vi "Read UUID.vi"(11 "UniqueName in":refnum<class "UniqueName.lvclass">) -> (2 "UUID":string, 3 "UniqueName out":refnum<class "UniqueName.lvclass">)   [LabVIEW 2014, in "UniqueName.lvlib" / "UniqueName.lvclass"]
uses:
  UniqueName.lvclass
  UniqueName.lvclass/UniqueName.ctl
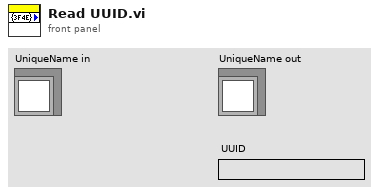
[diagram p1: front panel]
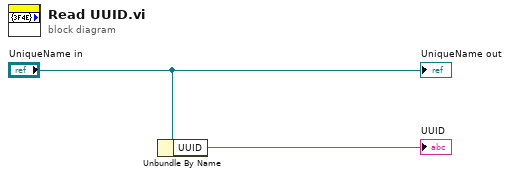
[diagram p0: block diagram]
diagram:
  n1 = Unbundle By Name("UniqueName in") -> ("UUID"=→"UUID":string)
  "UniqueName out" <- "UniqueName in"
